vi "Configure Current Output.vi"(0 "VISA resource name":refnum<visa-resource-name>, 1 "Enable Parallel Unit Sharing (False)":bool, 5 "Current Immediate Amplitude (0 A)":dbl, 7 "Current Triggered Amplitude (0 A)":dbl, 9 "Current Slew (Inf)":dbl=inf, 11 "error in (no error)":errorcluster, 12 "Enable Voltage Priority (False)":bool, 13 "Voltage Priority Current Lower Limit (-2.50A)":dbl=-2.5, 14 "Voltage Priority Current Upper Limit (2.50A)":dbl=2.5) -> (4 "VISA resource name out":refnum<visa-resource-name>, 15 "error out":errorcluster)   [LabVIEW 2022 SP3, in "Agilent N6900 N7900 Series.lvlib"]
doc: "Configures the output settings related to the current."
uses:
  Agilent N6900 N7900 Series.lvlib
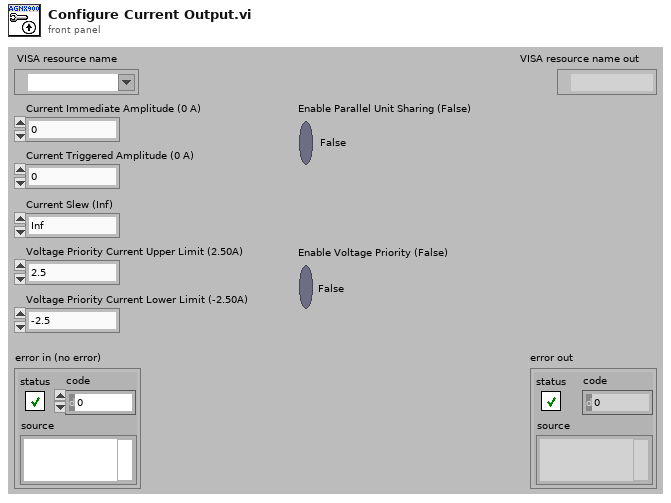
[diagram p1: front panel]
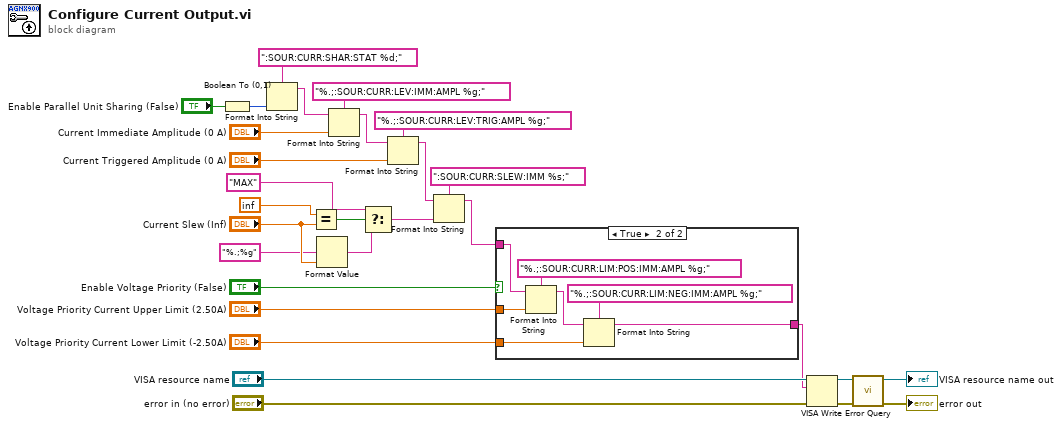
[diagram p0: block diagram]
diagram:
  n1 = Boolean To (0,1)(Boolean="Enable Parallel Unit Sharing (False)") -> (0, 1=w5:i16)
  n2 = Format Into String(format string=":SOUR:CURR:SHAR:STAT %d;", w5) -> (resulting string=w3:string)  [unwired: 2 in, 1 out]
  n3 = Equal?(x=inf, y="Current Slew (Inf)") -> (x = y?=w18:bool)
  n4 = Format Value(format string="%.;%g", value (0)="Current Slew (Inf)") -> (output string=w16:string)  [unwired: 1 in]
  n5 = Format Into String(format string="%.;:SOUR:CURR:LEV:IMM:AMPL %g;", initial string=w3, "Current Immediate Amplitude (0 A)") -> (resulting string=w8:string)  [unwired: 1 in, 1 out]
  n6 = Select(t="MAX", s=w18, f=w16) -> (s? t:f=w14:string)
  n7 = Format Into String(format string="%.;:SOUR:CURR:LEV:TRIG:AMPL %g;", initial string=w8, "Current Triggered Amplitude (0 A)") -> (resulting string=w1:string)  [unwired: 1 in, 1 out]
  n8 = Format Into String(format string=":SOUR:CURR:SLEW:IMM %s;", initial string=w1, w14) -> (resulting string=w20:string)  [unwired: 1 in, 1 out]
  n9 = case shown="True" "Enable Voltage Priority (False)" {
    tunnel: [w30 w37] -> w23
    tunnel: "Voltage Priority Current Lower Limit (-2.50A)" -> [_ w36]
    tunnel: "Voltage Priority Current Upper Limit (2.50A)" -> [_ w32]
    tunnel: w20 -> [w30 w31]
    frame False {
    }
    frame True {
      n10 = Format Into String(format string="%.;:SOUR:CURR:LIM:POS:IMM:AMPL %g;", initial string=w31, w32) -> (resulting string=w33:string)  [unwired: 1 in, 1 out]
      n11 = Format Into String(format string="%.;:SOUR:CURR:LIM:NEG:IMM:AMPL %g;", initial string=w33, w36) -> (resulting string=w37:string)  [unwired: 1 in, 1 out]
    }
  }
  n12 = VISA Write(VISA resource name="VISA resource name", write buffer=w23, error in (no error)="error in (no error)") -> (VISA resource name out=w26:refnum<visa-resource-name>, error out=w27:errorcluster)  [unwired: 1 out]
  n13 = call "Error Query.vi"("error in (no error)"=w27, "VISA resource name"=w26) -> ("error out"=→"error out":errorcluster, "VISA resource name out"=→"VISA resource name out":refnum<visa-resource-name>)  [unwired: 6 in, 2 out]
